vi "InsertIntoShortcutMenu.vi"(8 "error in":errorcluster, 9 "menu ref in":refnum<k9>, 11 "HW Engine in":refnum<class "HW Engine.lvclass">) -> (0 "error out":errorcluster, 1 "menu ref out":refnum<k9>, 3 "HW Engine out":refnum<class "HW Engine.lvclass">)   [LabVIEW 2025, in "HW Engine.lvlib" / "HW Engine.lvclass"]
doc: "Allows children to insert menu items without overriding ShortcutMenu.vi entirely. By default, called before Add/Remove.Copyright 2017 National Instruments Corporation\n\nLicensed under the Apache License, Version 2.0 (the \"License\"); you may not use this file except in compliance with the License. You may obtain a copy of the License at http://www.apache.org/licenses/LICENSE-2.0\nUnless required by applicable law or agreed to in writing, software distributed under the License is distributed on an \"AS IS\" BASIS, WITHOUT WARRANTIES OR CONDITIONS OF ANY KIND, either express or implied. See the License for the specific language governing permissions and limitations under the License."
uses:
  HW Engine.lvclass
  C:/Users/Public/Documents/Sandia National Labs/TSS Plugin/CEF.lvlibp/Node/CEF_Node.lvclass
  <vilib>/Utility/sysdir.llb/System Directory Type.ctl
  Users/Public/Documents/Sandia National Labs/TSS Plugin/CEF.lvlibp/Node/ReadChildren.vi
  Users/Public/Documents/Sandia National Labs/TSS Plugin/CEF.lvlibp/Node/ReadNodeClass.vi
  Users/Public/Documents/Sandia National Labs/TSS Plugin/CEF.lvlibp/Node/CEF_Node.lvclass
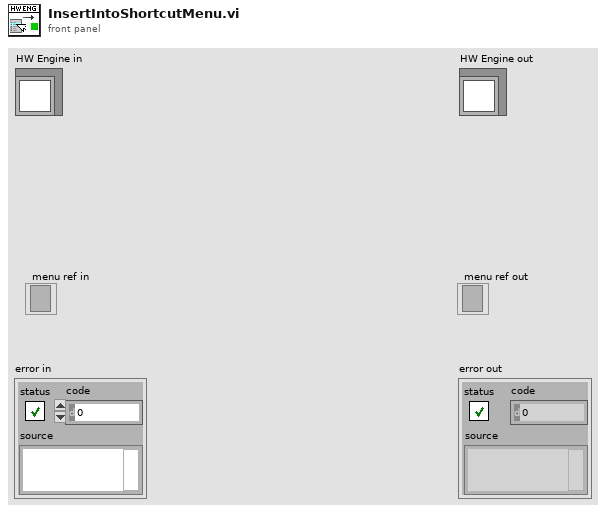
[diagram p1: front panel]
types:
  T1 = typedef "System Directory Type.ctl" = i32
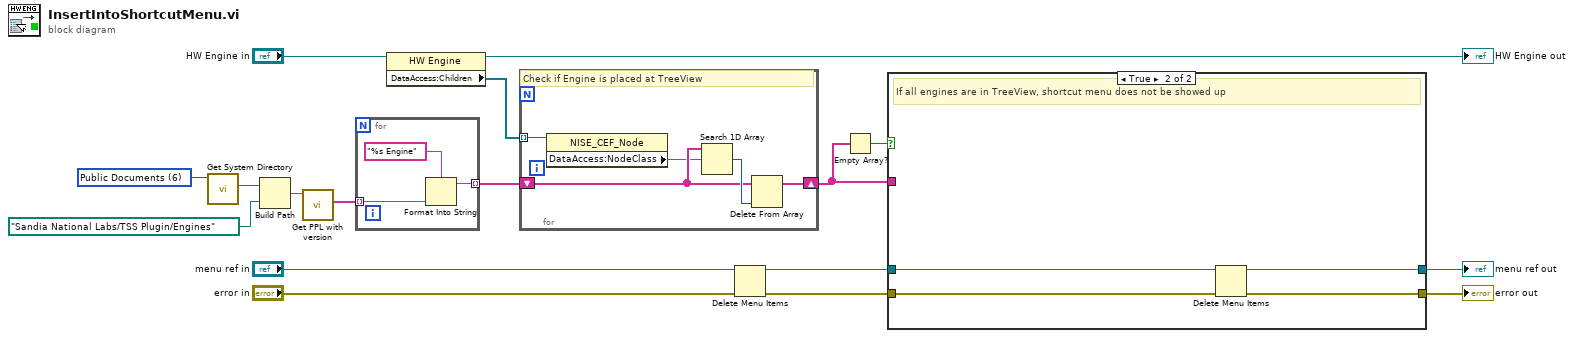
[diagram p0: block diagram]
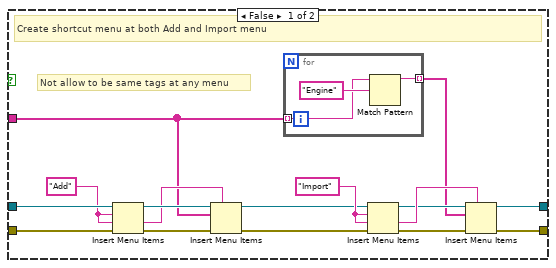
[diagram p2: hidden frame]
diagram:
  w4 = T1 6 items=["User Home"=0, "User Desktop"=1, "User Documents"=2, "User Application Data"=3, "User Preferences"=4, "User Temporary"=5, "Public Documents"=6, "Public Application Data"=7, "Public Preferences"=8, "Public Cache"=13, "System Core Libraries"=9, "System Installed Libraries"=10, "Application Files"=11, "Boot Volume Root"=12] ("system directory type")
  n1 = call <vilib>:"Get System Directory.vi"("system directory type"=w4) -> ("system directory"=w3:path)  [unwired: 10 in]
  n2 = Build Path(base path=w3, name or relative path=path "Sandia National Labs/TSS Plugin/Engines" ("PPL folder")) -> (appended path=w2:path)
  n3 = call "Get PPL with version.vi"("Plugin path"=w2) -> ("Plugin"=w1:string[])  [unwired: 9 in, 1 out]
  n4 = for {
    tunnel: [w20] -> w6 mode=indexing
    tunnel: w1 -> [w18] mode=indexing
    n5 = Format Into String(format string="%s Engine", w18) -> (resulting string=w20:string)  [unwired: 2 in, 1 out]
  }
  n6 = property class="HW Engine"(reference="HW Engine in") -> (reference out=→"HW Engine out":refnum<class "HW Engine.lvclass">, "DataAccess:Children"=w9:refnum<data-value>[])  [unwired: 1 in, 1 out]
  n7 = for {
    tunnel: w9 -> [w22] mode=indexing
    shift-right: [w23] -> w12
    shift-left: w6 -> [w24]
    # "Check if Engine is placed at TreeView"
    n8 = property class="NISE_CEF_Node"(reference=w22) -> ("DataAccess:NodeClass"=w21:string)  [unwired: 1 in, 2 out]
    n9 = Search 1D Array(1D array=w24, element=w21) -> (index of element=w25:i32)  [unwired: 1 in]
    n10 = Delete From Array(array=w24, index=w25) -> (array with subset deleted=w23:string[])  [unwired: 1 in, 1 out]
  }
  n11 = Delete Menu Items(6:"error in", 9:"menu ref in") -> (0:w15:errorcluster, 3:w14:refnum<k9>)  [unwired: 2 in]
  n12 = Empty Array?(array=w12) -> (empty?=w13:bool)
  n13 = case shown="True" w13 {
    tunnel: w15 -> [w41 w48]
    tunnel: [w29 w45] -> w8
    tunnel: w14 -> [w40 w46]
    tunnel: [w28 w47] -> w7
    tunnel: w12 -> [w27 _]
    frame False {
      w37 = "Add"
      w32 = "Import"
      # "Not allow to be same tags at any menu"
      # "Create shortcut menu at both Add and Import menu"
      n14 = Insert Menu Items(6:w41, 7:w37, 8:w37, 9:w40) -> (0:w38:errorcluster, 1:w36:string, 3:w39:refnum<k9>)  [unwired: 2 in]
      n15 = Insert Menu Items(5:w36, 6:w38, 8:w27, 9:w39) -> (0:w31:errorcluster, 3:w30:refnum<k9>)  [unwired: 2 in, 1 out]
      n16 = for {
        tunnel: w27 -> [w43] mode=indexing
        tunnel: [w42] -> w26 mode=indexing
        n17 = Match Pattern(string=w43, regular expression="Engine") -> (before substring=w42:string)  [unwired: 1 in, 3 out]
      }
      n18 = Insert Menu Items(6:w31, 7:w32, 8:w32, 9:w30) -> (0:w34:errorcluster, 1:w35:string, 3:w33:refnum<k9>)  [unwired: 2 in]
      n19 = Insert Menu Items(5:w35, 6:w34, 8:w26, 9:w33) -> (0:w28:errorcluster, 3:w29:refnum<k9>)  [unwired: 2 in, 1 out]
    }
    frame True {
      # "If all engines are in TreeView, shortcut menu does not be showed up"
      n20 = Delete Menu Items(6:w48, 9:w46) -> (0:w47:errorcluster, 3:w45:refnum<k9>)  [unwired: 2 in]
    }
  }
  "error out" <- w7
  "menu ref out" <- w8
